vi "signal_output.vi"(6 "acquire?":bool caption="Acquire?", 7 "pipeline counter in":u32, 8 "cluster in":T1) -> (1 "address bits out":u8, 2 "y data bits out":u8, 3 "x data bits out":u8)   [LabVIEW 2010]
uses:
  DDS_board_values_cluster.ctl
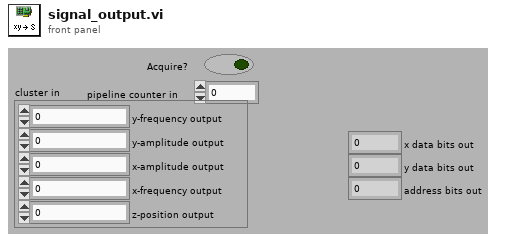
[diagram p1: front panel]
types:
  T1 = typedef "DDS_board_values_cluster.ctl" = cluster{"y-frequency output":fxp<+,36,32>, "y-amplitude output":u16, "x-amplitude output":u16, "x-frequency output":fxp<+,36,32>, "z-position output":i16}
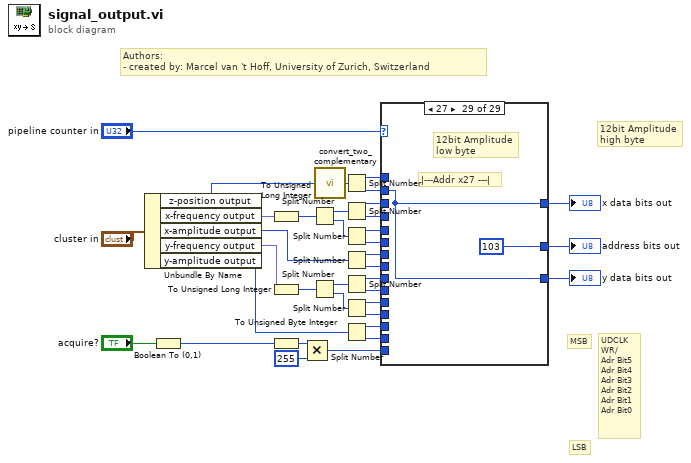
[diagram p0: block diagram]
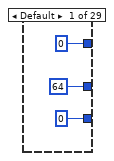
[diagram p2: hidden frame]
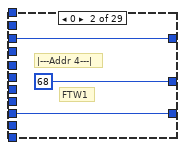
[diagram p3: hidden frame]
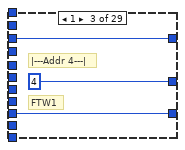
[diagram p4: hidden frame]
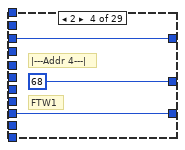
[diagram p5: hidden frame]
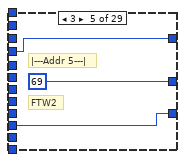
[diagram p6: hidden frame]
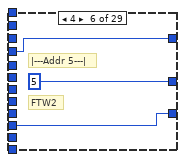
[diagram p7: hidden frame]
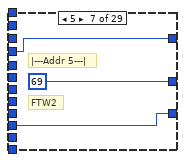
[diagram p8: hidden frame]
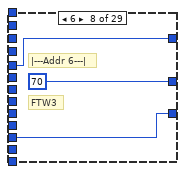
[diagram p9: hidden frame]
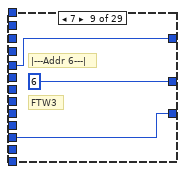
[diagram p10: hidden frame]
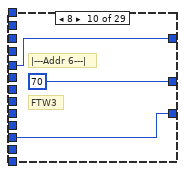
[diagram p11: hidden frame]
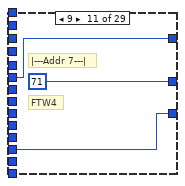
[diagram p12: hidden frame]
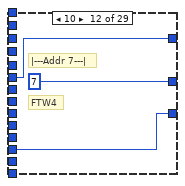
[diagram p13: hidden frame]
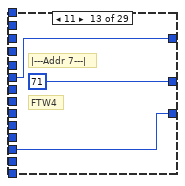
[diagram p14: hidden frame]
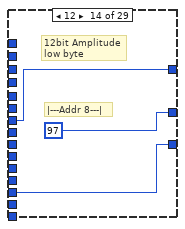
[diagram p15: hidden frame]
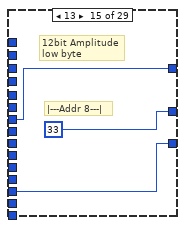
[diagram p16: hidden frame]
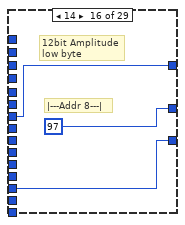
[diagram p17: hidden frame]
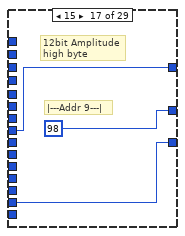
[diagram p18: hidden frame]
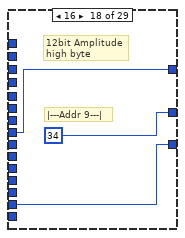
[diagram p19: hidden frame]
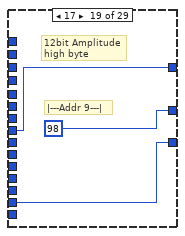
[diagram p20: hidden frame]
diagram:
  # "12bit Amplitude\nhigh byte"
  # "LSB"
  # "MSB"
  # "UDCLK\nWR/\nAdr Bit5\nAdr Bit4\nAdr Bit3\nAdr Bit2\nAdr Bit1\nAdr Bit0"
  # "Authors: \n- created by: Marcel van 't Hoff, University of Zurich, Switzerland"
  n1 = Unbundle By Name("cluster in") -> ("z-position output"=w4:i16, "x-frequency output"=w8:fxp<+,36,32>, "x-amplitude output"=w16:u16, "y-frequency output"=w7:fxp<+,36,32>, "y-amplitude output"=w15:u16)
  n2 = Boolean To (0,1)(Boolean="acquire?") -> (0, 1=w11:i16)
  n3 = To Unsigned Long Integer(number=w8) -> (unsigned 32bit integer=w6:u32)
  n4 = To Unsigned Long Integer(number=w7) -> (unsigned 32bit integer=w5:u32)
  n5 = To Unsigned Byte Integer(number=w11) -> (unsigned 8bit integer=w10:u8)
  n6 = Multiply(x=w10, y=u8 255) -> (x*y=w9:u8)
  n7 = Split Number(x=w6) -> (hi(x)=w18:u16, lo(x)=w19:u16)
  n8 = Split Number(x=w5) -> (hi(x)=w26:u16, lo(x)=w27:u16)
  n9 = call "convert_two_complementary.vi"("number in"=w4) -> ("complementary out"=w3:i16)  [unwired: 4 in]
  n10 = Split Number(x=w3) -> (hi(x)=w2:u8, lo(x)=w1:u8)
  n11 = Split Number(x=w18) -> (hi(x)=w20:u8, lo(x)=w21:u8)
  n12 = Split Number(x=w19) -> (hi(x)=w22:u8, lo(x)=w23:u8)
  n13 = Split Number(x=w16) -> (hi(x)=w32:u8, lo(x)=w33:u8)
  n14 = Split Number(x=w26) -> (hi(x)=w28:u8, lo(x)=w29:u8)
  n15 = Split Number(x=w27) -> (hi(x)=w30:u8, lo(x)=w31:u8)
  n16 = Split Number(x=w15) -> (hi(x)=w24:u8, lo(x)=w25:u8)
  n17 = case shown="27" "pipeline counter in" {
    tunnel: [u8 0 w42 w45 w48 w51 w54 w57 w60 w63 w66 w69 w72 w75 w76 w79 w82 w85 w88 w91 w95 w97 w99 w101 w102 w104 w106 w108 w110 w112] -> w34
    tunnel: w20 -> [_ w42 w45 w48 _ _ _ _ _ _ _ _ _ _ _ _ _ _ _ _ _ _ _ _ _ _ _ _ _]
    tunnel: w21 -> [_ _ _ _ w51 w54 w57 _ _ _ _ _ _ _ _ _ _ _ _ _ _ _ _ _ _ _ _ _ _]
    tunnel: w22 -> [_ _ _ _ _ _ _ w60 w63 w66 _ _ _ _ _ _ _ _ _ _ _ _ _ _ _ _ _ _ _]
    tunnel: w23 -> [_ _ _ _ _ _ _ _ _ _ w69 w72 w75 _ _ _ _ _ _ _ _ _ _ _ _ _ _ _ _]
    tunnel: w24 -> [_ _ _ _ _ _ _ _ _ _ _ _ _ w77 w80 w83 _ _ _ _ _ _ _ _ _ _ _ _ _]
    tunnel: w25 -> [_ _ _ _ _ _ _ _ _ _ _ _ _ _ _ _ w86 w89 w92 _ _ _ _ _ _ _ _ _ _]
    tunnel: w28 -> [_ w41 w44 w47 _ _ _ _ _ _ _ _ _ _ _ _ _ _ _ _ _ _ _ _ _ _ _ _ _]
    tunnel: w29 -> [_ _ _ _ w50 w53 w56 _ _ _ _ _ _ _ _ _ _ _ _ _ _ _ _ _ _ _ _ _ _]
    tunnel: w30 -> [_ _ _ _ _ _ _ w59 w62 w65 _ _ _ _ _ _ _ _ _ _ _ _ _ _ _ _ _ _ _]
    tunnel: w31 -> [_ _ _ _ _ _ _ _ _ _ w68 w71 w74 _ _ _ _ _ _ _ _ _ _ _ _ _ _ _ _]
    tunnel: [u8 0 w41 w44 w47 w50 w53 w56 w59 w62 w65 w68 w71 w74 w77 w80 w83 w86 w89 w92 w95 w97 w99 w101 w102 w104 w106 w108 w110 w112] -> w36
    tunnel: [u8 64 u8 68 u8 4 u8 68 u8 69 u8 5 u8 69 u8 70 u8 6 u8 70 u8 71 u8 7 u8 71 u8 97 u8 33 u8 97 u8 98 u8 34 u8 98 u8 99 u8 35 ("y") u8 35 ("y") u8 99 u8 102 u8 38 u8 102 u8 103 u8 39 u8 103] -> w35
    tunnel: w32 -> [_ _ _ _ _ _ _ _ _ _ _ _ _ w76 w79 w82 _ _ _ _ _ _ _ _ _ _ _ _ _]
    tunnel: w33 -> [_ _ _ _ _ _ _ _ _ _ _ _ _ _ _ _ w85 w88 w91 _ _ _ _ _ _ _ _ _ _]
    tunnel: w9 -> [_ _ _ _ _ _ _ _ _ _ _ _ _ _ _ _ _ _ _ w95 w97 w99 w101 _ _ _ _ _ _]
    tunnel: w2 -> [_ _ _ _ _ _ _ _ _ _ _ _ _ _ _ _ _ _ _ _ _ _ _ w102 w104 w106 _ _ _]
    tunnel: w1 -> [_ _ _ _ _ _ _ _ _ _ _ _ _ _ _ _ _ _ _ _ _ _ _ _ _ _ w108 w110 w112]
    frame Default {
    }
    frame 0 {
      # "FTW1"
      # "|---Addr 4---|"
    }
    frame 1 {
      # "FTW1"
      # "|---Addr 4---|"
    }
    frame 2 {
      # "FTW1"
      # "|---Addr 4---|"
    }
    frame 3 {
      # "FTW2"
      # "|---Addr 5---|"
    }
    frame 4 {
      # "FTW2"
      # "|---Addr 5---|"
    }
    frame 5 {
      # "FTW2"
      # "|---Addr 5---|"
    }
    frame 6 {
      # "FTW3"
      # "|---Addr 6---|"
    }
    frame 7 {
      # "FTW3"
      # "|---Addr 6---|"
    }
    frame 8 {
      # "FTW3"
      # "|---Addr 6---|"
    }
    frame 9 {
      # "FTW4"
      # "|---Addr 7---|"
    }
    frame 10 {
      # "FTW4"
      # "|---Addr 7---|"
    }
    frame 11 {
      # "FTW4"
      # "|---Addr 7---|"
    }
    frame 12 {
      # "12bit Amplitude\nlow byte"
      # "|---Addr 8---|"
    }
    frame 13 {
      # "12bit Amplitude\nlow byte"
      # "|---Addr 8---|"
    }
    frame 14 {
      # "12bit Amplitude\nlow byte"
      # "|---Addr 8---|"
    }
    frame 15 {
      # "12bit Amplitude\nhigh byte"
      # "|---Addr 9---|"
    }
    frame 16 {
      # "12bit Amplitude\nhigh byte"
      # "|---Addr 9---|"
    }
    frame 17 {
      # "12bit Amplitude\nhigh byte"
      # "|---Addr 9---|"
    }
    frame 18 {
      # "|---latch---|"
    }
    frame 19 {
      # "|---latch---|"
    }
    frame 20 {
      # "|---latch---|"
    }
    frame 21 {
      # "|---latch---|"
    }
    frame 22 {
      # "12bit Amplitude\nhigh byte"
      # "|---Addr x26 ---|"
    }
    frame 23 {
      # "12bit Amplitude\nhigh byte"
      # "|---Addr x26 ---|"
    }
    frame 24 {
      # "12bit Amplitude\nhigh byte"
      # "|---Addr x26 ---|"
    }
    frame 25 {
      # "12bit Amplitude\nlow byte"
      # "|---Addr x27 ---|"
    }
    frame 26 {
      # "12bit Amplitude\nlow byte"
      # "|---Addr x27 ---|"
    }
    frame 27 {
      # "12bit Amplitude\nlow byte"
      # "|---Addr x27 ---|"
    }
  }
  "y data bits out" <- w36
  "address bits out" <- w35
  "x data bits out" <- w34
